vi "ClearStandardEvents.vi"(8 "error in":errorcluster, 10 "standard events":T1, 11 "sub panel ref in":refnum<vi>) -> (0 "error out":errorcluster)   [LabVIEW 2025, in "CEF.lvlib"]
doc: "Copyright 2017 National Instruments Corporation\n\nLicensed under the Apache License, Version 2.0 (the \"License\"); you may not use this file except in compliance with the License. You may obtain a copy of the License at http://www.apache.org/licenses/LICENSE-2.0\nUnless required by applicable law or agreed to in writing, software distributed under the License is distributed on an \"AS IS\" BASIS, WITHOUT WARRANTIES OR CONDITIONS OF ANY KIND, either express or implied. See the License for the specific language governing permissions and limitations under the License."
uses:
  CEF.lvlib
  Node/StandardEvents.ctl
  Node/UserEventRef.ctl
  Controls/EventCluster.ctl
  Node/NodeChangeEvent.ctl
  Node/NodeRef.ctl
  Node/CEF_Node.lvclass
  Node/CacheState.ctl
  Node/RefreshUIEvent.ctl
  Node/StopEvent.ctl
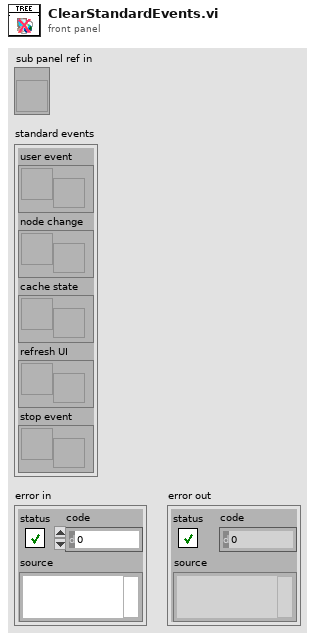
[diagram p1: front panel]
types:
  T1 = typedef "CEF.lvlib/CEF_Node.lvclass/StandardEvents.ctl" = cluster{"user event":T2, "node change":T3, "cache state":T4, "refresh UI":T5, "stop event":T6}
  T2 = typedef "CEF.lvlib/CEF_Node.lvclass/UserEventRef.ctl" = refnum<user-event>
  T3 = typedef "CEF.lvlib/CEF_Node.lvclass/NodeChangeEvent.ctl" = refnum<user-event>
  T4 = typedef "CEF.lvlib/CEF_Node.lvclass/CacheState.ctl" = refnum<user-event>
  T5 = typedef "CEF.lvlib/CEF_Node.lvclass/RefreshUIEvent.ctl" = refnum<user-event>
  T6 = typedef "CEF.lvlib/CEF_Node.lvclass/StopEvent.ctl" = refnum<user-event>
  T7 = typedef "CEF.lvlib/EventCluster.ctl" = cluster{"command":string, "data":string}
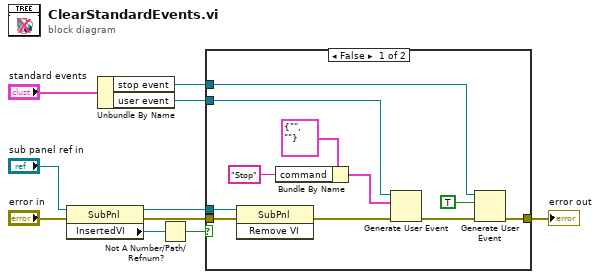
[diagram p0: block diagram]
diagram:
  n1 = property class="SubPnl"(reference="sub panel ref in", error in="error in") -> (reference out=w10:refnum<vi>, error out=w8:errorcluster, "InsertedVI"=w6:refnum<vi>)
  n2 = Unbundle By Name("standard events") -> ("stop event"=w1:T6, "user event"=w2:T2)
  n3 = Not A Number/Path/Refnum?(number/path/refnum=w6) -> (NaN/Path/Refnum?=w9:bool)
  n4 = case shown="False" w9 {
    tunnel: [w13 w22] -> w4
    tunnel: w10 -> [w21 _]
    tunnel: w8 -> [w19 w22]
    tunnel: w2 -> [w20 _]
    tunnel: w1 -> [w12 _]
    frame False {
      n5 = invoke class="SubPnl" method="Remove VI"(reference=w21, error in=w19) -> (error out=w18:errorcluster)  [unwired: 1 in, 2 out]
      n6 = Bundle By Name(cluster=T7 {"command"="", "data"=""} ("event data"), "command"="Stop") -> (w15:T7)
      n7 = Generate User Event(user event=w20, event data cluster=w15, error in=w18) -> (error out=w17:errorcluster)  [unwired: 1 in, 1 out]
      n8 = Generate User Event(user event=w12, event data cluster=TRUE ("event data"), error in=w17) -> (error out=w13:errorcluster)  [unwired: 1 in, 1 out]
    }
    frame True {
      # "Reference is not valid if there is no VI"
    }
  }
  "error out" <- w4
